vi "Control Type.vi"(11 "Valve in":refnum<class "BangBangControl.lvclass">) -> (2 "Valve Type":string)   [LabVIEW 2020, in "VolatusControl.lvlib" / "BangBangControl.lvclass"]
uses:
  BangBangControl.lvclass
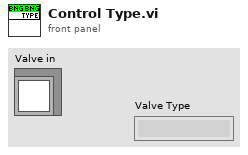
[diagram p1: front panel]
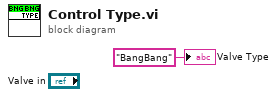
[diagram p0: block diagram]
diagram:
  "Valve Type" <- "BangBang" ("Valve Type")
